vi "_Export Data.vi"(7 "2D data":dbl[][](array[numeric]) format="%0.2f", 8 "file path (dialog if empty)":path) -> ()   [LabVIEW 2012]
doc: "Converts a 2D or 1D array of single-precision numbers to a text string and writes the string to a new byte stream file or appends the string to an existing file."
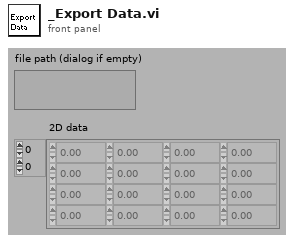
[diagram p1: front panel]
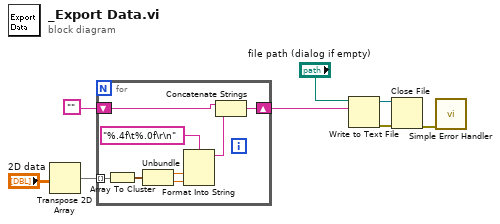
[diagram p0: block diagram]
diagram:
  n1 = Transpose 2D Array(2D array="2D data") -> (transposed array=w7:dbl[][])
  n2 = for {
    tunnel: w7 -> [w16] mode=indexing
    shift-right: [w11] -> w5
    shift-left: "" -> [w10]
    n3 = Array To Cluster(array=w16) -> (cluster=w15:cluster{"[0]":dbl, "[1]":dbl})
    n4 = Unbundle(w15) -> ("[0]"=w14:dbl, "[1]"=w13:dbl)
    n5 = Format Into String(format string="%.4f\t%.0f\r\n" ("format (%.3f)"), w14, w13) -> (resulting string=w9:string)  [unwired: 2 in, 1 out]
    n6 = Concatenate Strings(w10, w9) -> (w11:string)
  }
  n7 = Write to Text File(file (use dialog)="file path (dialog if empty)", text=w5) -> (refnum out=w2:refnum<file>, error out=w3:errorcluster)  [unwired: 2 in, 1 out]
  n8 = Close File(refnum=w2, error in=w3) -> (error out=w1:errorcluster)  [unwired: 1 out]
  n9 = call <vilib>:"Simple Error Handler.vi"("error in (no error)"=w1) -> ()  [unwired: 4 in, 5 out]
